vi "To String.vi"(8 "error in (no error)":errorcluster, 11 "BuildWorker Basics in":refnum<class "BuildWorker Basics.lvclass">) -> (0 "error out":errorcluster, 2 "String":string, 3 "BuildWorker Basics out":refnum<class "BuildWorker Basics.lvclass">)   [LabVIEW 2017, in "BuildWorker Controller.lvlib" / "BuildWorker Basics.lvclass"]
uses:
  BuildWorker Basics.lvclass
  BuildWorker Basics.lvclass/BuildWorker Basics.ctl
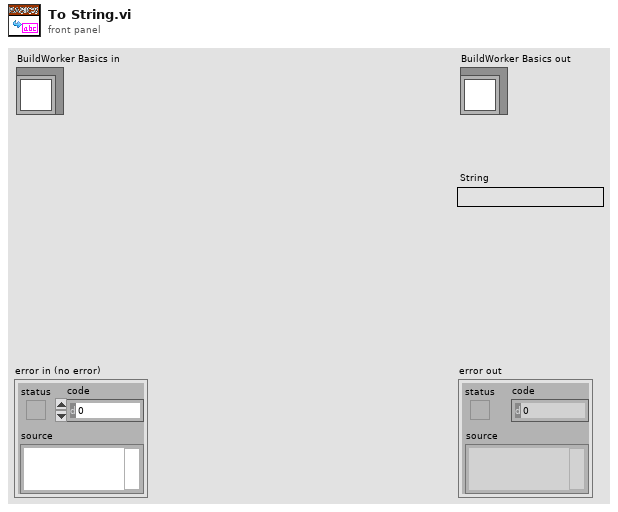
[diagram p1: front panel]
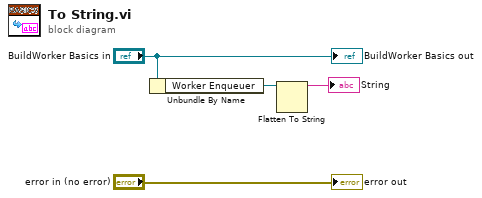
[diagram p0: block diagram]
diagram:
  n1 = Unbundle By Name("BuildWorker Basics in") -> ("Worker Enqueuer"=w2:refnum<class "Message Enqueuer.lvclass">)
  n2 = Flatten To String(anything=w2) -> (data string=→"String":string)  [unwired: 3 in, 2 out]
  "error out" <- "error in (no error)"
  "BuildWorker Basics out" <- "BuildWorker Basics in"
